vi "String Array Replace Local Decimal Separators 2D.vi"(1 "array in":string[][](array[string])) -> (0 "array out":string[][](array[string]))   [LabVIEW 2020]
doc: "This VI takes matrix of strings and tries to replace local decimal separators by dot."
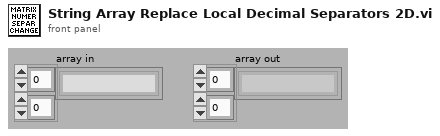
[diagram p1: front panel]
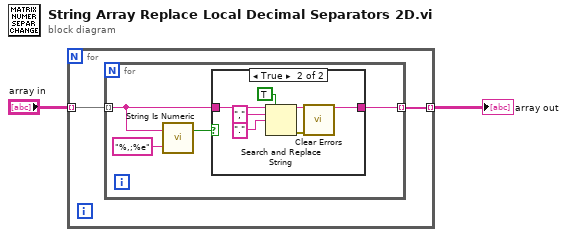
[diagram p0: block diagram]
diagram:
  n1 = for {
    tunnel: "array in" -> [w4] mode=indexing
    tunnel: [w3] -> w2 mode=indexing
    n2 = for {
      tunnel: w4 -> [w7] mode=indexing
      tunnel: [w8] -> w3 mode=indexing
      n3 = call "String Is Numeric.vi"("scan format (%.;%e)"="%,;%e" ("scan format (%.;)"), "String"=w7) -> ("is numeric"=w5:bool)  [unwired: 1 out]
      n4 = case shown="True" w5 {
        tunnel: [w9 w15] -> w8
        tunnel: w7 -> [w9 w10]
        frame False {
        }
        frame True {
          n5 = Search and Replace String(replace all?=TRUE ("replace all? (F)"), input string=w10, search string=",", replace string="." ("replace string (\"\")")) -> (result string=w15:string, error out=w11:errorcluster)  [unwired: 4 in, 2 out]
          n6 = call <vilib>:"Clear Errors.vi"("error in (no error)"=w11) -> ()  [unwired: 5 in, 2 out]
        }
      }
    }
  }
  "array out" <- w2
